vi "XY Graph Load Plot(s) Event.vi"(7 "Max Number of Plot to Load (-1: All)":i32=-1, 8 "Error In":errorcluster, 9 "File Path":path, 10 "Used Dialog? (T)":bool=TRUE, 11 "XYGraph Ref":T1) -> (0 "Error Out":errorcluster, 1 "Message":string, 2 "File Path(s)":path[](array[path]), 3 "Loaded Plot Names":cluster{"Plot Names":string[]}[](array[cluster]), 4 "# Plots Added":i32[](array[numeric]), 5 "Graph Name":string)   [LabVIEW 2019, in "XY Graph Add-Ons.lvlib"]
uses:
  XY Graph Add-Ons.lvlib
  XY Graph Refnum.ctl
  Files/ASCII File Header Definition.ctl
  <vilib>/Utility/error.llb/Error Cluster From Error Code.vi
  <vilib>/ErrorRing/Error Ring.xnode
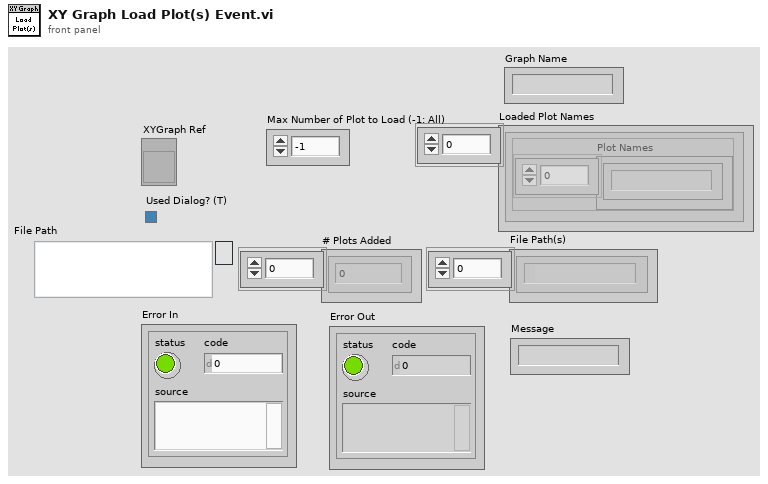
[diagram p1: front panel]
types:
  T1 = typedef "XY Graph Add-Ons.lvlib/XY Graph Refnum.ctl" = refnum<vi>
  T2 = typedef "ASCII File Header Definition.ctl" = cluster{"Number of Lines to Skip":i32, "Column Header Line?":bool}
  T3 = typedef "Plot Scale Labels.ctl" = cluster{"X Scale Label":string, "Y Scale Label":string}
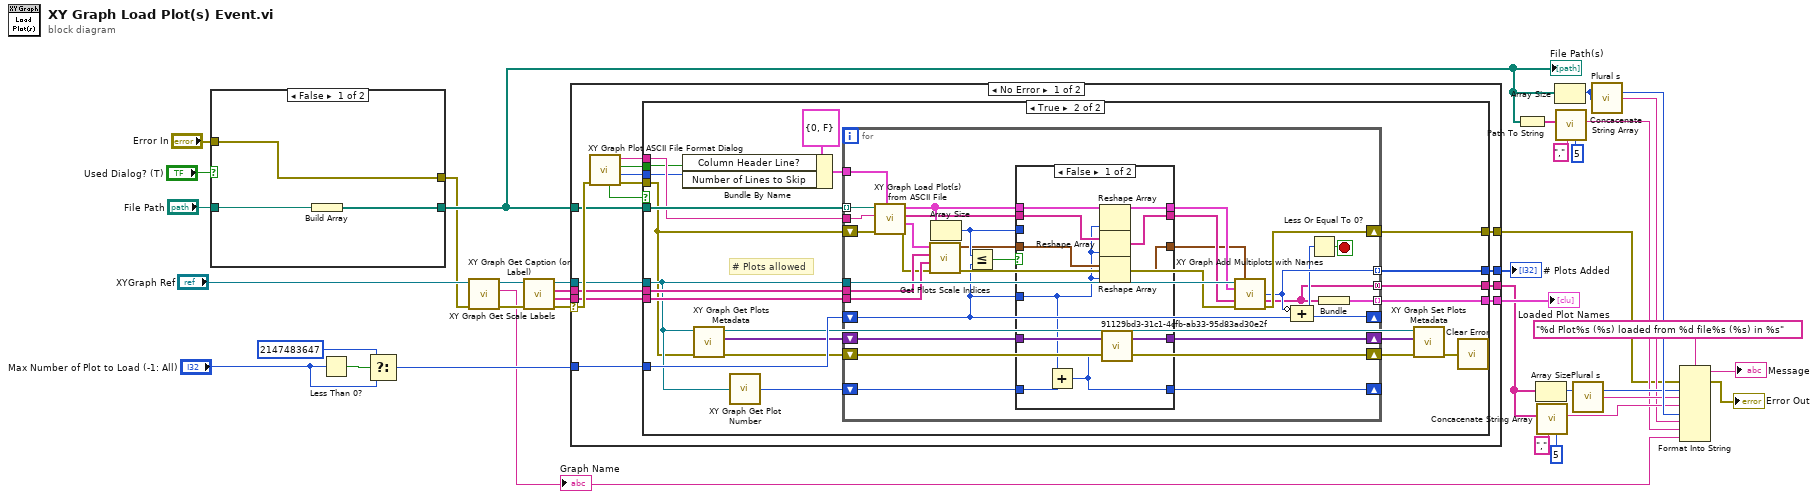
[diagram p0: block diagram]
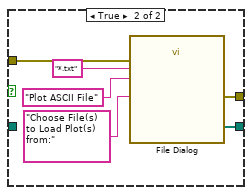
[diagram p2: hidden frame]
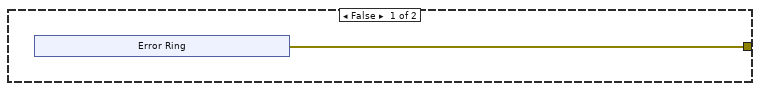
[diagram p3: hidden frame]
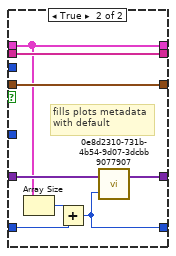
[diagram p4: hidden frame]
diagram:
  n1 = case shown="False" "Used Dialog? (T)" {
    tunnel: [w37 w41] -> w17
    tunnel: "Error In" -> [w36 w40]
    tunnel: [w36 w39] -> w4
    tunnel: "File Path" -> [w38 _]
    frame False {
      n2 = Build Array(w38) -> (w37:path[])
    }
    frame True {
      n3 = call "File Dialog"("prompt"="Choose File(s) to Load Plot(s) from:", "error in"=w40, "pattern (all files)"="*.txt", "pattern label"="Plot ASCII File") -> ("selected paths"=w41:path[], "error out"=w39:errorcluster)  [unwired: 8 in, 2 out]
    }
  }
  "File Path(s)" <- w17
  n4 = Less Than 0?(x="Max Number of Plot to Load (-1: All)") -> (x < 0?=w28:bool)
  n5 = Select(t=2147483647 ("Max Number of Plot to Load (-1: All)"), s=w28, f="Max Number of Plot to Load (-1: All)") -> (s? t:f=w25:i32)
  n6 = call "XY Graph Get Caption (or Label).vi"("error in (no error)"=w4, "XYGraph in"="XYGraph Ref") -> ("error out"=w9:errorcluster, "Caption (or Label) Text"=w8:string, "XYGraph out"=w34:T1)  [unwired: 7 in]
  "Graph Name" <- w8
  n7 = call "XY Graph Get Scale Labels.vi"("Error In"=w9, "XYGraph in"=w34) -> ("Error Out"=w3:errorcluster, "Y Scale Labels"=w31:string[], "X Scale Labels"=w32:string[], "XYGraph out"=w33:T1)  [unwired: 4 in, 2 out]
  n8 = case shown="No Error" w3 {
    selector: w3 -> [w59 w136]
    tunnel: w33 -> [w52 _]
    tunnel: w17 -> [w53 _]
    tunnel: [w51 _] -> w30
    tunnel: w32 -> [w50 _]
    tunnel: w31 -> [w49 _]
    tunnel: [w48 w136] -> w7
    tunnel: [w47 _] -> w29
    tunnel: w25 -> [w46 _]
    tunnel: [w45 _] -> w24
    frame No Error {
      n9 = call "XY Graph Plot ASCII File Format Dialog.vi"("error in (no error)"=w59) -> ("error out"=w57:errorcluster, "Number of Lines to Skip"=w54:i32, "Column Header Line?"=w55:bool, "Separator"=w56:string, "OK"=w58:bool)  [unwired: 6 in]
      n10 = case shown="True" w58 {
        tunnel: w57 -> [_ w65]
        tunnel: w56 -> [_ w84]
        tunnel: w55 -> [_ w83]
        tunnel: w54 -> [_ w82]
        tunnel: w53 -> [_ w85]
        tunnel: w52 -> [_ w71]
        tunnel: [_ w86] -> w51
        tunnel: w50 -> [_ w79]
        tunnel: w49 -> [_ w78]
        tunnel: [w60 w77] -> w48
        tunnel: [_ w76] -> w47
        tunnel: w46 -> [_ w75]
        tunnel: [_ w74] -> w45
        frame False {
          n11 = xnode "Error Ring"() -> ("error out"=w60:errorcluster)
        }
        frame True {
          # "# Plots allowed"
          n12 = Bundle By Name(cluster=T2 {"Number of Lines to Skip"=0, "Column Header Line?"=FALSE} ("Header Definitions"), "Column Header Line?"=w83, "Number of Lines to Skip"=w82) -> (w80:T2)
          n13 = call "XY Graph Get Plots Metadata.vi"("Error In"=w65, "XYGraph Ref"=w71) -> ("Error Out"=w73:errorcluster, "Plots Metadata"=w72:variant[], "XYGraph Ref (dup)"=w67:T1)  [unwired: 6 in, 1 out]
          n14 = call "XY Graph Get Plot Number.vi"("XYGraph"=w71) -> ("# Plots"=w70:i32)  [unwired: 8 in]
          n15 = for {
            tunnel: w71 -> [w116]
            tunnel: [w106] -> w86 mode=indexing
            tunnel: w85 -> [w115] mode=indexing
            tunnel: w84 -> [w113]
            tunnel: w80 -> [w112]
            tunnel: w79 -> [w111]
            tunnel: w78 -> [w110]
            shift-right: [w105] -> w77
            shift-left: w65 -> [w114]
            tunnel: [w99] -> w76 mode=indexing
            shift-right: [w98] -> _
            shift-left: w75 -> [w93]
            tunnel: [w92] -> w74 mode=concatenating
            shift-right: [w88] -> w69
            shift-left: w73 -> [w88]
            shift-right: [w89] -> w66
            shift-left: w72 -> [w91]
            shift-right: [w87] -> _
            shift-left: w70 -> [w90]
            stop <- w97 stop-if-true
            n16 = call "XY Graph Load Plot(s) from ASCII File.vi"("Header Definitions"=w112, "error in (no error)"=w114, "Delimiter (TAB)"=w113, "File Path"=w115) -> ("error out"=w108:errorcluster, "Plot Scales Array"=w109:T3[], "Plot Name Array"=w101:string[], "Plot Array"=w102:cluster{"X Array":dbl[], "Y Array":dbl[]}[])  [unwired: 3 in, 1 out]
            n17 = call "Get Plots Scale Indices.vi"("Error In"=w108, "Y Scale Labels"=w110, "X Scale Labels"=w111, "Plot Scales Array"=w109) -> ("Error Out"=w107:errorcluster, "Array of Scales (Default)"=w100:cluster{"X Scale":u32, "Y Scale":u32}[])  [unwired: 6 in]
            n18 = Array Size(array=w102) -> (size(s)=w103:i32)
            n19 = Less Or Equal?(x=w103, y=w93) -> (x <= y?=w104:bool)
            n20 = case shown="False" w104 {
              tunnel: w103 -> [_ _]
              tunnel: w102 -> [w127 w132]
              tunnel: w101 -> [w123 w135]
              tunnel: w100 -> [w125 w134]
              tunnel: [w126 w132] -> w96
              tunnel: [w122 w135] -> w95
              tunnel: [w124 w134] -> w94
              tunnel: w93 -> [w118 _]
              tunnel: w91 -> [w121 w133]
              tunnel: w90 -> [w119 w130]
              tunnel: [w120 w129] -> w89
              tunnel: [w117 w128] -> w87
              frame False {
                n21 = Add(x=w118, y=w119) -> (x+y=w117:i32)
                n22 = Reshape Array(w127, w118) -> (w126:cluster{"X Array":dbl[], "Y Array":dbl[]}[])
                n23 = Reshape Array(w123, w118) -> (w122:string[])
                n24 = Reshape Array(w125, w118) -> (w124:cluster{"X Scale":u32, "Y Scale":u32}[])
                n25 = call "91129bd3-31c1-4cfb-ab33-95d83ad30e2f.vi"("dimension size"=w117, "1D Array"=w121) -> ("1D Array"=w120:variant[])  [unwired: 1 in]
              }
              frame True {
                # "fills plots metadata\nwith default"
                n26 = Array Size(array=w132) -> (size(s)=w131:i32)
                n27 = Add(x=w131, y=w130) -> (x+y=w128:i32)
                n28 = call "0e8d2310-731b-4b54-9d07-3dcbb9077907.vi"("dimension size"=w128, "1D Array"=w133) -> ("1D Array"=w129:variant[])  [unwired: 1 in]
              }
            }
            n29 = call "XY Graph Add Multiplots with Names.vi"("XYGraph in"=w116, "Array of Scales (Default)"=w94, "Array of Plots"=w96, "Array of Plot Names (\"Plot\")"=w95, "error in (no error)"=w107) -> ("Number of Plots Added"=w99:i32, "Added Plot Names"=w92:string[], "error out"=w105:errorcluster)  [unwired: 6 in, 2 out]
            n30 = Compound Arithmetic op=ADD(invert w99, w93) -> (w98:i32)
            n31 = Less Or Equal To 0?(x=w98) -> (x <= 0?=w97:bool)
            n32 = Bundle("Added Plot Names"=w92) -> (w106:cluster{"Added Plot Names":string[]})  [unwired: 1 in]
          }
          n33 = call "XY Graph Set Plots Metadata.vi"("error in (no error)"=w69, "Plots Metadata"=w66, "XY Graph Refnum"=w67) -> ("error out"=w68:errorcluster)  [unwired: 7 in, 1 out]
          n34 = call "Clear Error.vi"("Error In"=w68) -> ()  [unwired: 8 in, 1 out]
        }
      }
    }
    frame Error {
    }
  }
  "Loaded Plot Names" <- w30
  "# Plots Added" <- w29
  n35 = Path To String(path=w17) -> (string=w18:string[])
  n36 = Array Size(array=w24) -> (size(s)=w14:i32)
  n37 = call "Concacenate String Array.vi"("Max Number of Elements (None: -1)"=5 ("Max Number of Elements (None: 1)"), "Separator (TAB)"=",", "String Array"=w24) -> ("Formatted String"=w12:string)  [unwired: 8 in]
  n38 = Array Size(array=w17) -> (size(s)=w15:i32)
  n39 = call "Concacenate String Array.vi"("Max Number of Elements (None: -1)"=5 ("Max Number of Elements (None: 1)"), "Separator (TAB)"=",", "String Array"=w18) -> ("Formatted String"=w11:string)  [unwired: 8 in]
  n40 = call "Plural s.vi"("# Elements"=w14) -> ("Plural s"=w13:string)
  n41 = call "Plural s.vi"("# Elements"=w15) -> ("Plural s"=w10:string)
  n42 = Format Into String(format string="%d Plot%s (%s) loaded from %d file%s (%s) in %s", error in=w7, w14, w13, w12, w15, w10, w11, w8) -> (resulting string=→"Message":string, error out=→"Error Out":errorcluster)  [unwired: 1 in]
